vi "Configure FPGA Write.vi"(8 "Error In":errorcluster, 11 "Draw Frame In":refnum<class "Draw Frame.lvclass">) -> (0 "Error Out":errorcluster, 3 "Draw Frame Out":refnum<class "Draw Frame.lvclass">)   [LabVIEW 2019, in "Draw Frame.lvclass"]
uses:
  Draw Frame.lvclass
  Accessors/Display/Get Display.vi
  Accessors/FPGA Reference/Get FPGA Reference.vi
  <vilib>/Memosfet/myRIO-Neopixel/RT/Display/Display.lvclass
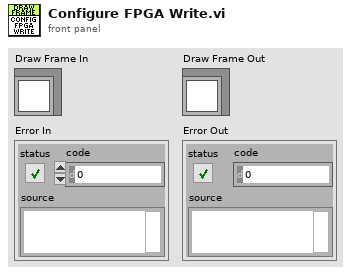
[diagram p1: front panel]
types:
  T1 = typedef "Draw Frame.lvclass/FPGA Reference.ctl" = refnum<k20>
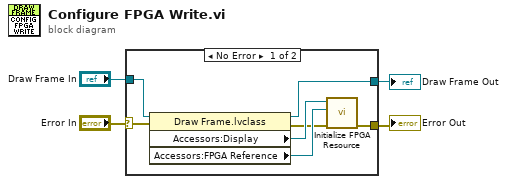
[diagram p0: block diagram]
diagram:
  n1 = case shown="No Error" "Error In" {
    selector: "Error In" -> [w9 w12]
    tunnel: [w5 w12] -> w4
    tunnel: [w11 w13] -> w3
    tunnel: "Draw Frame In" -> [w10 w13]
    frame No Error {
      n2 = property class="Draw Frame.lvclass"(reference=w10, error in=w9) -> (reference out=w11:refnum<class "Draw Frame.lvclass">, error out=w6:errorcluster, "Accessors:Display"=w7:refnum<class "Display.lvclass">, "Accessors:FPGA Reference"=w8:T1)
      n3 = call <vilib>:"Initialize FPGA Resource.vi"("Error In"=w6, "FPGA VI Reference"=w8, "Display In"=w7) -> ("Error Out"=w5:errorcluster)  [unwired: 7 in, 1 out]
    }
    frame Error {
    }
  }
  "Error Out" <- w4
  "Draw Frame Out" <- w3
